vi "New Image.vi"(8 "error in (no error)":errorcluster, 9 "Buffer Number":i32, 10 "Image":T1, 11 "IMAQ Display in":refnum<class "HIJ Vision File Viewer.lvclass">) -> (0 "error out":errorcluster, 3 "IMAQ Display out":refnum<class "HIJ Vision File Viewer.lvclass">)   [LabVIEW 2014, in "HIJ Vision File Viewer.lvlib" / "HIJ Vision File Viewer.lvclass"]
uses:
  HIJ Vision File Viewer.lvclass
  Display Actors/HIJ Vision Display/HIJ Vision Display/HIJ Vision Display.lvclass
  <vilib>/vision/Image Controls.llb/IMAQ Image.ctl
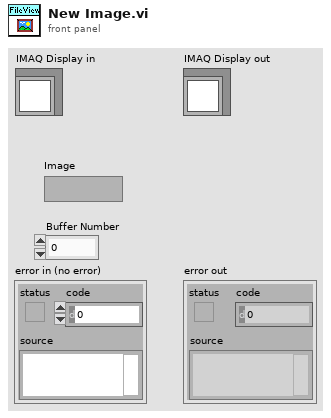
[diagram p1: front panel]
types:
  T1 = typedef "IMAQ Image.ctl" = refnum<image>
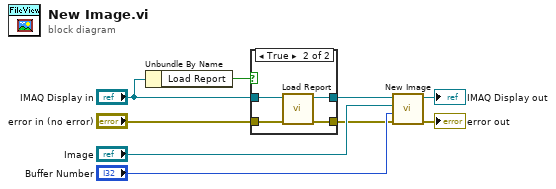
[diagram p0: block diagram]
diagram:
  n1 = Unbundle By Name("IMAQ Display in") -> ("Load Report"=w1:bool)
  n2 = case shown="True" w1 {
    tunnel: "IMAQ Display in" -> [w11 w15]
    tunnel: [w11 w14] -> w5
    tunnel: "error in (no error)" -> [w10 w13]
    tunnel: [w10 w12] -> w3
    frame False {
    }
    frame True {
      n3 = call-dynamic "Load Report.vi"("error in (no error)"=w13, "HIJ Vision File Viewer in"=w15) -> ("error out"=w12:errorcluster, "HIJ Vision File Viewer out"=w14:refnum<class "HIJ Vision File Viewer.lvclass">)  [unwired: 8 in]
    }
  }
  n4 = call-parent "New Image.vi"("error in (no error)"=w3, "Buffer Number"="Buffer Number", "Image"="Image", "IMAQ Display in"=w5) -> ("error out"=→"error out":errorcluster, "IMAQ Display out"=→"IMAQ Display out":refnum<class "HIJ Vision File Viewer.lvclass">)  [unwired: 6 in]
